vi "Calculate FPGA Parameters.vi"(5 "Accumulator Size (bit)":i32=32, 6 "Amplitude Scaling Parameters":T1={"Full Scale (V) "=10.0, "Full Scale (binary)"=32768.0}, 7 "Loop Rate (Hz)":dbl, 9 "Signal Amplitude (V)":dbl=5.0, 10 "Phase Shift (Deg)":dbl, 11 "DDS Signal Frequency (Hz)":dbl=20000.0) -> (0 "Scaling Ratio":dbl, 1 "AO Amplitude":u16, 2 "Phase Shift":u32, 3 "Accumulator Increment":u32)   [LabVIEW 2017]
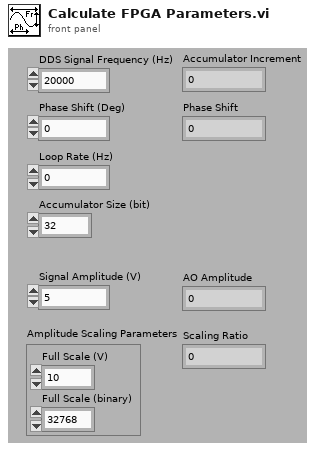
[diagram p1: front panel]
types:
  T1 = cluster{"Full Scale (V) ":dbl, "Full Scale (binary)":dbl}
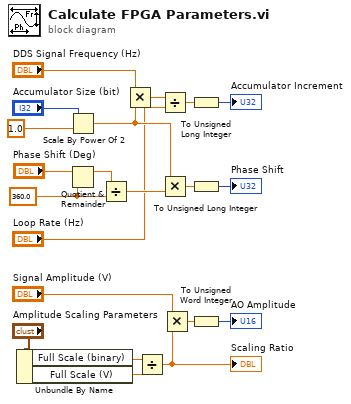
[diagram p0: block diagram]
diagram:
  w1 = 360.0 ("y")
  n1 = Unbundle By Name("Amplitude Scaling Parameters") -> ("Full Scale (binary)"=w7:dbl, "Full Scale (V)"=w6:dbl)
  n2 = Scale By Power Of 2(n="Accumulator Size (bit)", x=1.0) -> (x*2^n=w13:dbl)
  n3 = Quotient & Remainder(x="Phase Shift (Deg)", y=w1) -> (x-y*floor(x/y)=w2:dbl)  [unwired: 1 out]
  n4 = Divide(x=w2, y=w1) -> (x/y=w16:dbl)
  n5 = Multiply(x="DDS Signal Frequency (Hz)", y=w13) -> (x*y=w15:dbl)
  n6 = Divide(x=w7, y=w6) -> (x/y=w5:dbl)
  "Scaling Ratio" <- w5
  n7 = Divide(x=w15, y="Loop Rate (Hz)") -> (x/y=w20:dbl)
  n8 = Multiply(x=w13, y=w16) -> (x*y=w10:dbl)
  n9 = Multiply(x="Signal Amplitude (V)", y=w5) -> (x*y=w12:dbl)
  n10 = To Unsigned Long Integer(number=w20) -> (unsigned 32bit integer=→"Accumulator Increment":u32)
  n11 = To Unsigned Long Integer(number=w10) -> (unsigned 32bit integer=→"Phase Shift":u32)
  n12 = To Unsigned Word Integer(number=w12) -> (unsigned 16bit integer=→"AO Amplitude":u16)
